vi "GC EX CMS Vacuum - Step 2.vi"(7 "Step":i32, 8 "error in":errorcluster, 9 "Test Results In":T8, 10 "Gas":T1, 11 "GC Configuration":T2) -> (0 "error out":errorcluster, 1 "Test Results Out":T8, 2 "Gas Out":T1 caption="Gas", 3 "GC Configuration Out":T2)   [LabVIEW 2015]
uses:
  Controls/Test Information.ctl
  Controls/Vacuum Test.ctl
  Controls/Test Timing.ctl
  Controls/Vaccum Thresholds.ctl
  Controls/Helium Test.ctl
  Controls/Helium Thresholds.ctl
  CAN Communication/Gas/Typedefs/Session Handle.ctl
  CAN Communication/Gas/Gas.lvclass
  Controls/Test Results.ctl
  Controls/Step Result.ctl
  CAN Communication/Gas/Typedefs/Valves.ctl
  SubVIs/Timing/Timing.lvlib
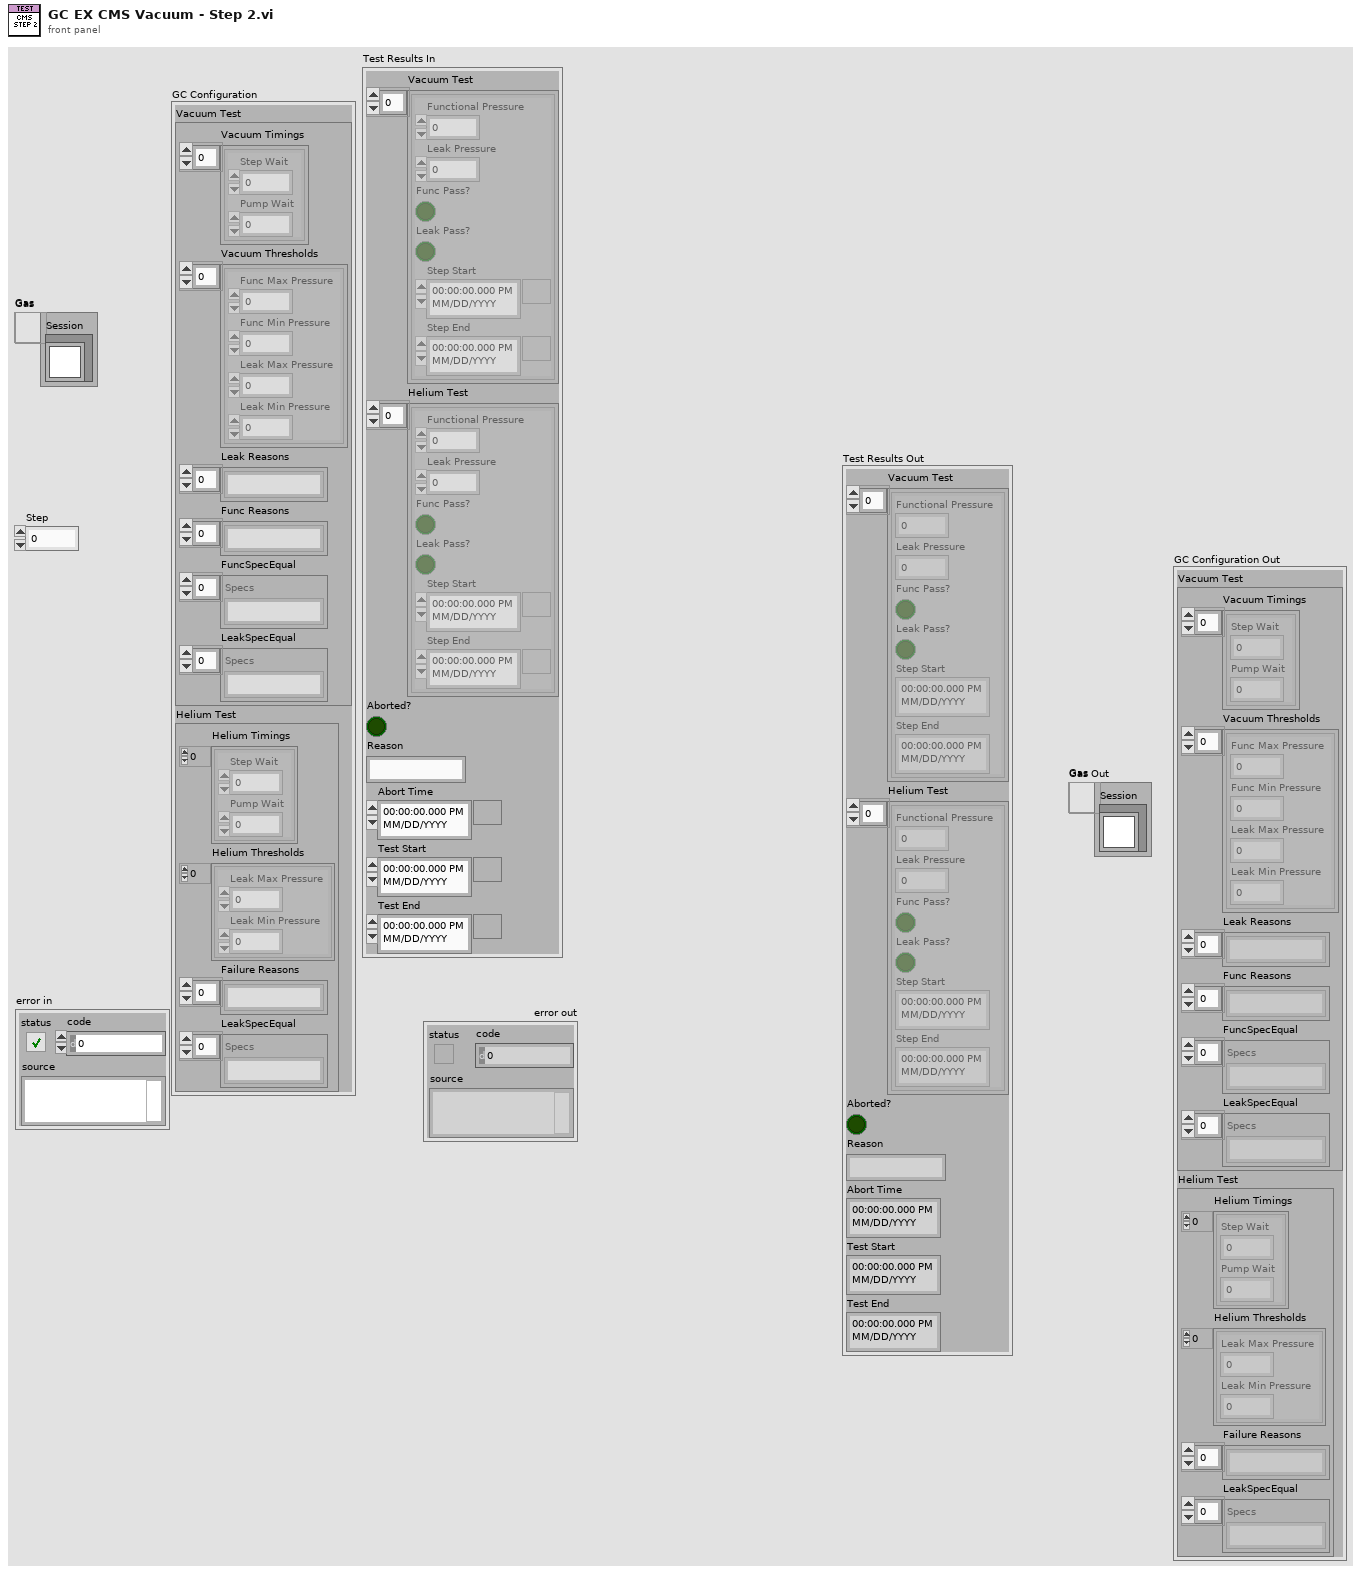
[diagram p1: front panel]
types:
  T1 = typedef "Gas.lvclass/Session Handle.ctl" = refnum<data-value>
  T2 = typedef "Test Information.ctl" = cluster{"Vacuum Test":T3, "Helium Test":T6}
  T3 = typedef "Vacuum Test.ctl" = cluster{"Vacuum Timings":T4[], "Vacuum Thresholds":T5[], "Leak Reasons":string[], "Func Reasons":string[], "FuncSpecEqual":string[], "LeakSpecEqual":string[]}
  T4 = typedef "Test Timing.ctl" = cluster{"Step Wait":dbl, "Pump Wait":dbl}
  T5 = typedef "Vaccum Thresholds.ctl" = cluster{"Func Max Pressure":dbl, "Func Min Pressure":dbl, "Leak Max Pressure":dbl, "Leak Min Pressure":dbl}
  T6 = typedef "Helium Test.ctl" = cluster{"Helium Timings":T4[], "Helium Thresholds":T7[], "Failure Reasons":string[], "LeakSpecEqual":string[]}
  T7 = typedef "Helium Thresholds.ctl" = cluster{"Leak Max Pressure":dbl, "Leak Min Pressure":dbl}
  T8 = typedef "Test Results.ctl" = cluster{"Vacuum Test":T9[], "Helium Test":T9[], "Aborted?":bool, "Reason":string, "Abort Time":timestamp, "Test Start":timestamp, "Test End":timestamp}
  T9 = typedef "Step Result.ctl" = cluster{"Functional Pressure":dbl, "Leak Pressure":dbl, "Func Pass?":bool, "Leak Pass?":bool, "Step Start":timestamp, "Step End":timestamp}
  T10 = typedef "Gas.lvclass/Valves.ctl" = u16
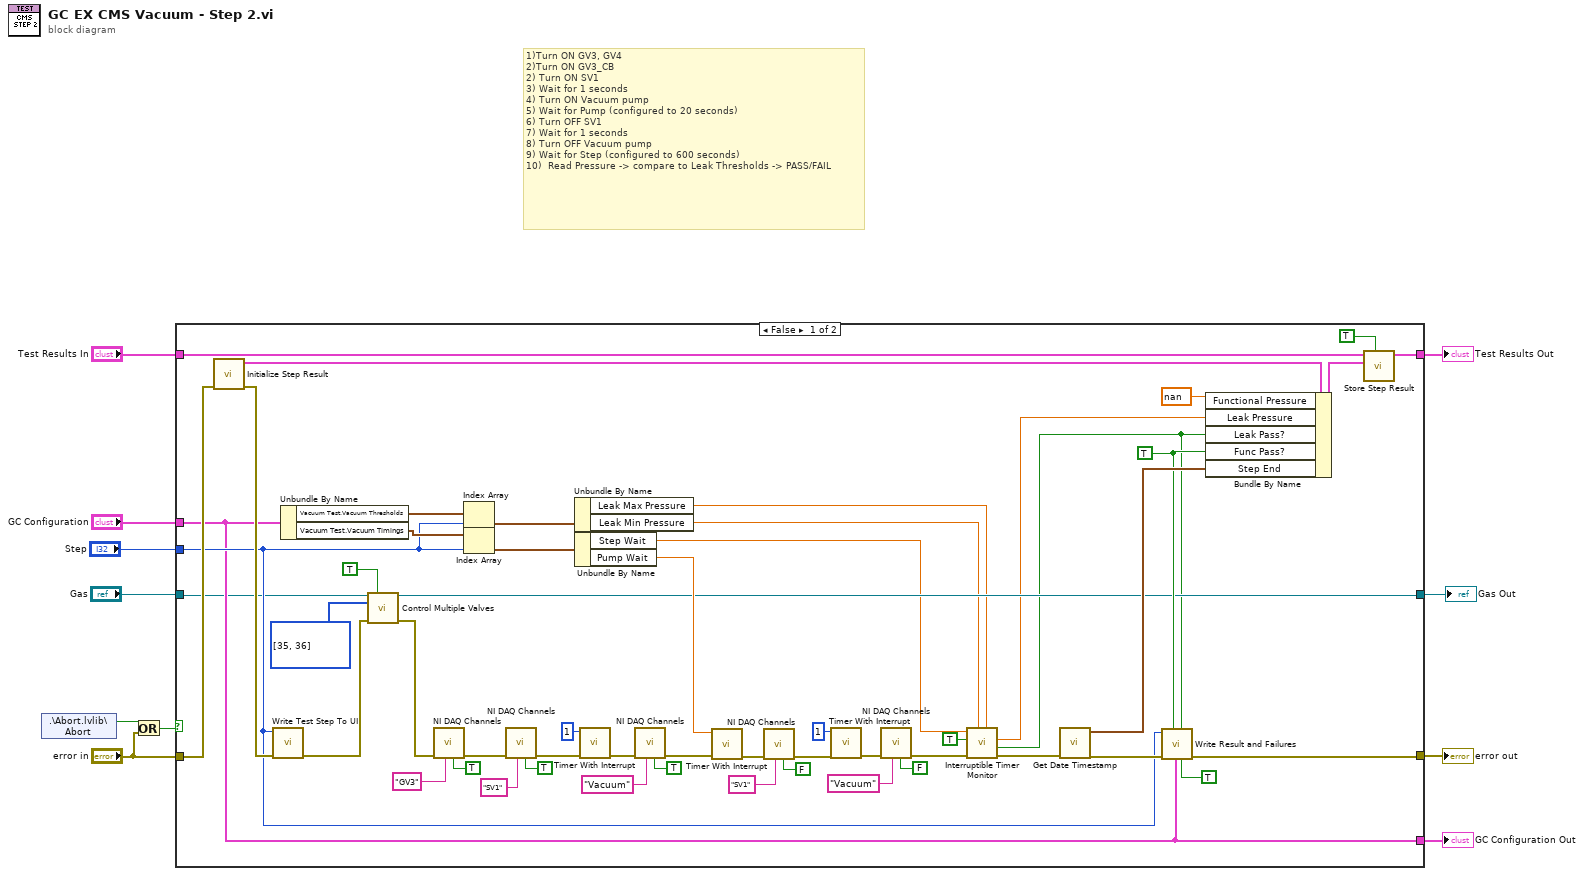
[diagram p0: block diagram]
diagram:
  # "1)Turn ON GV3, GV4\n2)Turn ON GV3_CB\n2) Turn ON SV1\n3) Wait for 1 seconds\n4) Turn ON Vacuum pump\n5) Wait for Pump (configured to 20 seconds)\n6) Turn OFF SV1\n7) Wait for 1 seconds\n8) Turn OFF Vacuum pump\n9) Wait for Step (configured to 600 seconds)\n10)  Read Pressure -> compare to Leak Thresholds -> PASS/FAIL"
  n1 = shared-variable ".\\Abort.lvlib\\Abort"() -> (w10:bool)  [unwired: 1 in, 1 out]
  n2 = Or(x=w10, y="error in") -> (x .or. y?=w9:bool)
  n3 = case shown="False" w9 {
    tunnel: "error in" -> [w64 w67]
    tunnel: "Test Results In" -> [w61 w68]
    tunnel: [w62 w68] -> w7
    tunnel: [w52 w67] -> w6
    tunnel: "GC Configuration" -> [w50 w66]
    tunnel: "Step" -> [w51 _]
    tunnel: [w50 w66] -> w3
    tunnel: [w40 w65] -> w1
    tunnel: "Gas" -> [w46 w65]
    frame False {
      w41 = TRUE ("Func Pass?")
      w45 = T10[] [35, 36] items=["GV1"=33, "GV2"=34, "GV3"=35, "GV4"=36, "GV5"=37, "GV6"=38, "GV7"=39, "GV8"=40, "GV9"=41, "GV10"=42, "GV11"=43, "LV3"=51, "LV4"=52] ("Valves")
      n4 = call "Initialize Step Result.vi"("error in (no error)"=w64) -> ("error out"=w63:errorcluster, "New Step Result"=w60:T9)  [unwired: 8 in, 1 out]
      n5 = call "Write Test Step To UI.vi"("error in (no error)"=w63, "Step"=w51) -> ("error out"=w43:errorcluster)  [unwired: 9 in]
      n6 = Unbundle By Name(w50) -> ("Vacuum Test.Vacuum Thresholds"=w57:T5[], "Vacuum Test.Vacuum Timings"=w56:T4[])
      n7 = call "Control Multiple Valves.vi"("Session Handle in"=w46, "Energize?"=TRUE, "Valves"=w45, "error in (no error)"=w43) -> ("Session Handle out"=w40:T1, "error out"=w37:errorcluster)  [unwired: 8 in, 2 out]
      n8 = call "NI DAQ Channels.vi"("Control"=TRUE ("State"), "Channel"="GV3", "error in (no error)"=w37) -> ("error out"=w35:errorcluster)  [unwired: 7 in, 1 out]
      n9 = Index Array(array=w57, index=w51) -> (element=w54:T5)
      n10 = Index Array(array=w56, index=w51) -> (element=w55:T4)
      n11 = call "NI DAQ Channels.vi"("Control"=TRUE ("State"), "Channel"="SV1", "error in (no error)"=w35) -> ("error out"=w34:errorcluster)  [unwired: 7 in, 1 out]
      n12 = Unbundle By Name(w54) -> ("Leak Max Pressure"=w20:dbl, "Leak Min Pressure"=w21:dbl)
      n13 = Unbundle By Name(w55) -> ("Step Wait"=w23:dbl, "Pump Wait"=w48:dbl)
      n14 = call "Timer With Interrupt.vi"("error in (no error)"=w34, "Wait (s)"=1) -> ("error out"=w32:errorcluster)  [unwired: 7 in, 2 out]
      n15 = call "NI DAQ Channels.vi"("Control"=TRUE ("State"), "Channel"="Vacuum", "error in (no error)"=w32) -> ("error out"=w31:errorcluster)  [unwired: 7 in, 1 out]
      n16 = call "Timer With Interrupt.vi"("error in (no error)"=w31, "Wait (s)"=w48) -> ("error out"=w29:errorcluster)  [unwired: 7 in, 2 out]
      n17 = call "NI DAQ Channels.vi"("Control"=FALSE ("State"), "Channel"="SV1", "error in (no error)"=w29) -> ("error out"=w28:errorcluster)  [unwired: 7 in, 1 out]
      n18 = call "Timer With Interrupt.vi"("error in (no error)"=w28, "Wait (s)"=1) -> ("error out"=w26:errorcluster)  [unwired: 7 in, 2 out]
      n19 = call "NI DAQ Channels.vi"("Control"=FALSE ("State"), "Channel"="Vacuum", "error in (no error)"=w26) -> ("error out"=w24:errorcluster)  [unwired: 7 in, 1 out]
      n20 = call "Interruptible Timer Monitor.vi"("Max"=w20, "Min"=w21, "error in (no error)"=w24, "Update UI?"=TRUE, "Wait (s)"=w23) -> ("error out"=w18:errorcluster, "In Range?"=w17:bool, "Leak Rate"=w19:dbl)  [unwired: 2 in, 2 out]
      n21 = call "Get Date Timestamp.vi"("error in (no error)"=w18) -> ("error out"=w53:errorcluster, "current time"=w58:timestamp)  [unwired: 9 in]
      n22 = call "Write Result and Failures.vi"("Vacuum?"=TRUE, "Leak"=w17, "GC Configuration"=w50, "Func"=w41, "error in (no error)"=w53, "Step"=w51) -> ("error out"=w52:errorcluster)  [unwired: 5 in]
      n23 = Bundle By Name(cluster=w60, "Functional Pressure"=nan, "Leak Pressure"=w19, "Leak Pass?"=w17, "Func Pass?"=w41, "Step End"=w58) -> (w59:T9)
      n24 = call "Store Step Result.vi"("Vacuum?"=TRUE, "Step Result"=w59, "Test Results In"=w61) -> ("Test Results Out"=w62:T8)  [unwired: 8 in]
    }
    frame True {
    }
  }
  "error out" <- w6
  "Test Results Out" <- w7
  "GC Configuration Out" <- w3
  "Gas Out" <- w1
